vi "test_F9P_fgv-ver.vi"() -> ()   [LabVIEW 2019] (continued)
,2,13,08,65,355,35,09,07,194,,10,16,222,19,11,37,142,,3*73\r\n$GBGSV,4,3,13,13,50,315,36,14,76,037,37,28,59,310,,33,73,239,,3*78\r\n$GBGSV,4,4,13,34,13,142,,3*44\r\n$GNGLL,3723.61864,N,12656.97538,E,064330.00,A,A*7B\r\n$GNRMC,064331.00,A,3723.61873,N,12656.97627,E,2.634,76.09,250720,,,A,V*35\r\n$GNVTG,76.09,T,,M,2.634,N,4.879,K,A*1A\r\n$GNGGA,064331.00,3723.61873,N,12656.97627,E,1,12,0.67,43.8,M,18.5,M,,*75\r\n$GNGSA,A,3,17,19,06,12,05,02,09,,,,,,1.19,0.67,0.98,1*0D\r\n$GNGSA,A,3,85,70,71,72,,,,,,,,,1.19,0.67,0.98,2*02\r\n$GNGSA,A,3,36,19,11,04,09,12,,,,,,,1.19,0.67,0.98,3*09\r\n$GNGSA,A,3,28,14,13,33,08,10,,,,,,,1.19,0.67,0.98,4*09\r\n$GPGSV,4,1,13,02,66,335,45,04,08,037,40,05,48,262,42,06,58,077,45,1*6A\r\n$GPGSV,4,2,13,07,06,104,,09,38,057,48,12,18,263,,13,08,191,19,1*6E\r\n$GPGSV,4,3,13,17,19,158,28,19,37,161,33,25,11,294,20,29,07,323,16,1*60\r\n$GPGSV,4,4,13,30,01,134,,1*52\r\n$GPGSV,4,1,13,02,66,335,,04,08,037,39,05,48,262,37,06,58,077,39,6*6B\r\n$GPGSV,4,2,13,07,06,104,,09,38,057,42,12,18,263,12,13,08,191,,6*68\r\n$GPGSV,4,3,13,17,19,158,28,19,37,161,,25,11,294,,29,07,323,,6*62\r\n$GPGSV,4,4,13,30,01,134,,6*55\r\n$GLGSV,2,1,06,70,54,030,29,71,69,224,39,72,18,217,28,84,08,134,08,1*7C\r\n$GLGSV,2,2,06,85,63,113,37,86,52,337,,1*7F\r\n$GLGSV,2,1,06,70,54,030,,71,69,224,28,72,18,217,20,84,08,134,11,3*75\r\n$GLGSV,2,2,06,85,63,113,28,86,52,337,,3*73\r\n$GAGSV,3,1,09,02,04,287,08,04,68,085,43,09,44,196,25,11,78,037,40,7*74\r\n$GAGSV,3,2,09,12,32,115,29,18,55,284,40,19,17,042,31,25,01,241,,7*7F\r\n$GAGSV,3,3,09,36,35,314,22,7*4F\r\n$GAGSV,3,1,09,02,04,287,,04,68,085,39,09,44,196,22,11,78,037,32,2*76\r\n$GAGSV,3,2,09,12,32,115,25,18,55,284,43,19,17,042,31,25,01,241,,2*75\r\n$GAGSV,3,3,09,36,35,314,22,2*4A\r\n$GBGSV,4,1,13,04,35,133,,05,09,257,,06,27,182,,07,09,201,,1*7B\r\n$GBGSV,4,2,13,08,65,355,41,09,07,194,,10,16,222,19,11,37,142,,1*72\r\n$GBGSV,4,3,13,13,50,315,39,14,76,037,44,28,59,310,42,33,73,239,41,1*72\r\n$GBGSV,4,4,13,34,13,142,23,1*47\r\n$GBGSV,4,1,13,04,35,133,,05,09,257,,06,27,182,,07,09,201,17,3*7F\r\n$GBGSV,4,2,13,08,65,355,36,09,07,194,,10,16,222,19,11,37,142,,3*70\r\n$GBGSV,4,3,13,13,50,315,38,14,76,037,39,28,59,310,,33,73,239,,3*78\r\n$GBGSV,4,4,13,34,13,142,,3*44\r\n$GNGLL,3723.61873,N,12656.97627,E,064331.00,A,A*71\r\n$GNRMC,064332.00,A,3723.61883,N,12656.97715,E,2.685,76.91,250720,,,A,V*32\r\n$GNVTG,76.91,T,,M,2.685,N,4.973,K,A*1A\r\n$GNGGA,064332.00,3723.61883,N,12656.97715,E,1,12,0.67,43.7,M,18.5,M,,*76\r\n$GNGSA,A,3,17,19,06,12,05,02,09,,,,,,1.19,0.67,0.98,1*0D\r\n$GNGSA,A,3,85,70,71,72,,,,,,,,,1.19,0.67,0.98,2*02\r\n$GNGSA,A,3,36,19,11,04,09,12,,,,,,,1.19,0.67,0.98,3*09\r\n$GNGSA,A,3,28,34,14,13,33,08,10,,,,,,1.19,0.67,0.98,4*0E\r\n$GPGSV,4,1,13,02,66,335,45,04,08,037,27,05,48,262,43,06,58,077,43,1*6C\r\n$GPGSV,4,2,13,07,06,104,,09,38,057,45,12,18,263,,13,08,191,22,1*6B\r\n$GPGSV,4,3,13,17,19,158,33,19,37,161,28,25,11,294,19,29,07,323,17,1*6B\r\n$GPGSV,4,4,13,30,01,134,,1*52\r\n$GPGSV,4,1,13,02,66,335,,04,08,037,37,05,48,262,38,06,58,077,38,6*6B\r\n$GPGSV,4,2,13,07,06,104,,09,38,057,43,12,18,263,11,13,08,191,,6*6A\r\n$GPGSV,4,3,13,17,19,158,29,19,37,161,,25,11,294,,29,07,323,,6*63\r\n$GPGSV,4,4,13,30,01,134,,6*55\r\n$GLGSV,2,1,06,70,54,030,36,71,69,224,40,72,18,217,30,84,08,134,09,1*74\r\n$GLGSV,2,2,06,85,63,113,30,86,52,337,,1*78\r\n$GLGSV,2,1,06,70,54,030,,71,69,224,28,72,18,217,20,84,08,134,11,3*75\r\n$GLGSV,2,2,06,85,63,113,28,86,52,337,,3*73\r\n$GAGSV,3,1,09,02,04,287,10,04,68,085,40,09,44,196,32,11,78,037,38,7*77\r\n$GAGSV,3,2,09,12,32,115,29,18,55,284,41,19,17,042,33,25,01,241,,7*7C\r\n$GAGSV,3,3,09,36,35,314,24,7*49\r\n$GAGSV,3,1,09,02,04,287,,04,68,085,35,09,44,196,29,11,78,037,31,2*72\r\n$GAGSV,3,2,09,12,32,115,25,18,55,284,44,19,17,042,37,25,01,241,,2*74\r\n$GAGSV,3,3,09,36,35,314,22,2*4A\r\n$GBGSV,4,1,13,04,35,133,,05,09,257,,06,27,182,,07,09,201,,1*7B\r\n$GBGSV,4,2,13,08,65,355,41,09,07,194,,10,16,222,19,11,37,142,,1*72\r\n$GBGSV,4,3,13,13,50,315,39,14,76,037,42,28,59,310,43,33,73,239,41,1*75\r\n$GBGSV,4,4,13,34,13,142,25,1*41\r\n$GBGSV,4,1,13,04,35,133,,05,09,257,,06,27,182,,07,09,201,13,3*7B\r\n$GBGSV,4,2,13,08,65,355,36,09,07,194,,10,16,222,21,11,37,142,,3*7B\r\n$GBGSV,4,3,13,13,50,315,35,14,76,037,37,28,59,310,,33,73,239,,3*7B\r\n$GBGSV,4,4,13,34,13,142,,3*44\r\n$GNGLL,3723.61883,N,12656.97715,E,064332.00,A,A*7D\r\n$GNRMC,064333.00,A,3723.61900,N,12656.97803,E,2.812,70.91,250720,,,A,V*37\r\n$GNVTG,70.91,T,,M,2.812,N,5.207,K,A*15\r\n$GNGGA,064333.00,3723.61900,N,12656.97803,E,1,12,0.67,43.7,M,18.5,M,,*75\r\n$GNGSA,A,3,17,19,06,05,02,09,,,,,,,1.18,0.67,0.98,1*0F\r\n$GNGSA,A,3,85,70,71,72,,,,,,,,,1.18,0.67,0.98,2*03\r\n$GNGSA,A,3,36,19,11,04,09,12,,,,,,,1.18,0.67,0.98,3*08\r\n$GNGSA,A,3,28,11,14,13,33,08,10,,,,,,1.18,0.67,0.98,4*08\r\n$GPGSV,4,1,13,02,66,335,44,04,08,037,37,05,48,262,42,06,58,077,46,1*68\r\n$GPGSV,4,2,13,07,06,104,,09,38,057,45,12,18,263,,13,08,191,21,1*68\r\n$GPGSV,4,3,13,17,19,158,29,19,37,161,32,25,11,294,20,29,07,323,15,1*63\r\n$GPGSV,4,4,13,30,01,134,,1*52\r\n$GPGSV,4,1,13,02,66,335,,04,08,037,37,05,48,262,38,06,58,077,37,6*64\r\n$GPGSV,4,2,13,07,06,104,,09,38,057,43,12,18,263,,13,08,191,,6*6A\r\n$GPGSV,4,3,13,17,19,158,26,19,37,161,,25,11,294,,29,07,323,,6*6C\r\n$GPGSV,4,4,13,30,01,134,,6*55\r\n$GLGSV,2,1,06,70,54,030,35,71,69,224,42,72,18,217,30,84,08,134,15,1*78\r\n$GLGSV,2,2,06,85,63,113,41,86,52,337,,1*7E\r\n$GLGSV,2,1,06,70,54,030,,71,69,224,27,72,18,217,19,84,08,134,10,3*71\r\n$GLGSV,2,2,06,85,63,113,28,86,52,337,,3*73\r\n$GAGSV,3,1,09,02,04,287,08,04,68,085,43,09,44,196,36,11,78,037,40,7*76\r\n$GAGSV,3,2,09,12,32,115,31,18,55,284,41,19,17,042,34,25,01,241,,7*72\r\n$GAGSV,3,3,09,36,35,314,24,7*49\r\n$GAGSV,3,1,09,02,04,287,,04,68,085,37,09,44,196,33,11,78,037,33,2*79\r\n$GAGSV,3,2,09,12,32,115,24,18,55,284,45,19,17,042,37,25,01,241,,2*74\r\n$GAGSV,3,3,09,36,35,314,23,2*4B\r\n$GBGSV,4,1,13,04,35,133,,05,09,257,,06,27,182,,07,09,201,,1*7B\r\n$GBGSV,4,2,13,08,65,355,41,09,07,194,,10,16,222,18,11,37,142,30,1*70\r\n$GBGSV,4,3,13,13,50,315,40,14,76,037,44,28,59,310,42,33,73,239,42,1*7F\r\n$GBGSV,4,4,13,34,13,142,,1*46\r\n$GBGSV,4,1,13,04,35,133,,05,09,257,,06,27,182,,07,09,201,14,3*7C\r\n$GBGSV,4,2,13,08,65,355,38,09,07,194,,10,16,222,20,11,37,142,,3*74\r\n$GBGSV,4,3,13,13,50,315,38,14,76,037,37,28,59,310,,33,73,239,,3*76\r\n$GBGSV,4,4,13,34,13,142,,3*44\r\n$GNGLL,3723.61900,N,12656.97803,E,064333.00,A,A*7E\r\n$GNRMC,064334.00,A,3723.61923,N,12656.97890,E,2.813,67.43,250720,,,A,V*33\r\n$GNVTG,67.43,T,,M,2.813,N,5.210,K,A*1B\r\n$GNGGA,064334.00,3723.61923,N,12656.97890,E,1,12,0.66,43.6,M,18.5,M,,*79\r\n$GNGSA,A,3,17,19,06,05,02,09,,,,,,,1.18,0.66,0.98,1*0E\r\n$GNGSA,A,3,85,70,71,72,,,,,,,,,1.18,0.66,0.98,2*02\r\n$GNGSA,A,3,36,19,11,04,09,12,,,,,,,1.18,0.66,0.98,3*09\r\n$GNGSA,A,3,28,11,14,13,33,08,10,,,,,,1.18,0.66,0.98,4*09\r\n$GPGSV,4,1,13,02,66,335,43,04,08,037,33,05,48,262,41,06,58,077,49,1*67\r\n$GPGSV,4,2,13,07,06,104,,09,38,057,40,12,18,263,,13,08,191,20,1*6C\r\n$GPGSV,4,3,13,17,19,158,34,19,37,161,28,25,11,294,20,29,07,323,16,1*67\r\n$GPGSV,4,4,13,30,01,134,,1*52\r\n$GPGSV,4,1,13,02,66,335,,04,08,037,32,05,48,262,37,06,58,077,32,6*6B\r\n$GPGSV,4,2,13,07,06,104,,09,38,057,40,12,18,263,,13,08,191,,6*69\r\n$GPGSV,4,3,13,17,19,158,31,19,37,161,,25,11,294,,29,07,323,,6*6A\r\n$GPGSV,4,4,13,30,01,134,,6*55\r\n$GLGSV,2,1,06,70,54,030,27,71,69,224,42,72,18,217,30,84,08,134,12,1*7C\r\n$GLGSV,2,2,06,85,63,113,43,86,52,337,,1*7C\r\n$GLGSV,2,1,06,70,54,030,,71,69,224,28,72,18,217,19,84,08,134,10,3*7E\r\n$GLGSV,2,2,06,85,63,113,27,86,52,337,,3*7C\r\n$GAGSV,3,1,09,02,04,287,11,04,68,085,45,09,44,196,38,11,78,037,38,7*79\r\n$GAGSV,3,2,09,12,32,115,25,18,55,284,38,19,17,042,34,25,01,241,,7*79\r\n$GAGSV,3,3,09,36,35,314,25,7*48\r\n$GAGSV,3,1,09,02,04,287,,04,68,085,37,09,44,196,36,11,78,037,35,2*7A\r\n$GAGSV,3,2,09,12,32,115,24,18,55,284,44,19,17,042,35,25,01,241,,2*77\r\n$GAGSV,3,3,09,36,35,314,23,2*4B\r\n$GBGSV,4,1,13,04,35,133,,05,09,257,,06,27,182,,07,09,201,,1*7B\r\n$GBGSV,4,2,13,08,65,355,41,09,07,194,,10,16,222,18,11,37,142,34,1*74\r\n$GBGSV,4,3,13,13,50,315,39,14,76,037,44,28,59,310,41,33,73,239,42,1*72\r\n$GBGSV,4,4,13,34,13,142,,1*46\r\n$GBGSV,4,1,13,04,35,133,,05,09,257,,06,27,182,,07,09,201,,3*79\r\n$GBGSV,4,2,13,08,65,355,38,09,07,194,,10,16,222,21,11,37,142,,3*75\r\n$GBGSV,4,3,13,13,50,315,39,14,76,037,38,28,59,310,,33,73,239,,3*78\r\n$GBGSV,4,4,13,34,13,142,,3*44\r\n$GNGLL,3723.61923,N,12656.97890,E,064334.00,A,A*72\r\n$GNRMC,064335.00,A,3723.61955,N,12656.97980,E,3.032,64.24,250720,,,A,V*3B\r\n$GNVTG,64.24,T,,M,3.032,N,5.615,K,A*12\r\n$GNGGA,064335.00,3723.61955,N,12656.97980,E,1,12,0.66,44.0,M,18.5,M,,*78\r\n$GNGSA,A,3,17,19,06,05,02,09,,,,,,,1.18,0.66,0.98,1*0E\r\n$GNGSA,A,3,85,70,71,72,,,,,,,,,1.18,0.66,0.98,2*02\r\n$GNGSA,A,3,36,19,11,04,09,12,,,,,,,1.18,0.66,0.98,3*09\r\n$GNGSA,A,3,28,11,14,13,33,08,10,,,,,,1.18,0.66,0.98,4*09\r\n$GPGSV,4,1,13,02,66,335,40,04,08,037,30,05,48,262,41,06,58,077,49,1*67\r\n$GPGSV,4,2,13,07,06,104,,09,38,057,42,12,18,262,,13,08,191,20,1*6F\r\n$GPGSV,4,3,13,17,19,158,32,19,37,161,29,25,11,294,20,29,07,323,16,1*60\r\n$GPGSV,4,4,13,30,01,134,,1*52\r\n$GPGSV,4,1,13,02,66,335,,04,08,037,35,05,48,262,35,06,58,077,35,6*69\r\n$GPGSV,4,2,13,07,06,104,,09,38,057,43,12,18,262,,13,08,191,,6*6B\r\n$GPGSV,4,3,13,17,19,158,27,19,37,161,,25,11,294,,29,07,323,,6*6D\r\n$GPGSV,4,4,13,30,01,134,,6*55\r\n$GLGSV,2,1,06,70,54,030,32,71,69,224,42,72,18,217,29,84,08,134,09,1*7A\r\n$GLGSV,2,2,06,85,63,113,40,86,52,337,,1*7F\r\n$GLGSV,2,1,06,70,54,030,,71,69,224,29,72,18,217,20,84,08,134,15,3*70\r\n$GLGSV,2,2,06,85,63,113,26,86,52,337,,3*7D\r\n$GAGSV,3,1,09,02,04,287,08,04,68,085,45,09,44,196,38,11,78,037,39,7*70\r\n$GAGSV,3,2,09,12,32,115,35,18,55,284,39,19,17,042,39,25,01,241,,7*74\r\n$GAGSV,3,3,09,36,35,314,24,7*49\r\n$GAGSV,3,1,09,02,04,287,,04,68,085,37,09,44,196,34,11,78,037,32,2*7F\r\n$GAGSV,3,2,09,12,32,115,22,18,55,284,44,19,17,042,34,25,01,241,,2*70\r\n$GAGSV,3,3,09,36,35,314,23,2*4B\r\n$GBGSV,4,1,13,04,35,133,,05,09,257,,06,27,182,,07,09,201,,1*7B\r\n$GBGSV,4,2,13,08,65,355,40,09,07,194,,10,16,222,21,11,37,142,29,1*73\r\n$GBGSV,4,3,13,13,50,315,39,14,76,037,44,28,59,310,41,33,73,239,42,1*72\r\n$GBGSV,4,4,13,34,13,142,,1*46\r\n$GBGSV,4,1,13,04,35,133,,05,09,257,,06,27,182,,07,09,201,,3*79\r\n$GBGSV,4,2,13,08,65,355,38,09,07,194,,10,16,222,21,11,37,142,28,3*7F\r\n$GBGSV,4,3,13,13,50,315,37,14,76,037,39,28,59,310,,33,73,239,,3*77\r\n$GBGSV,4,4,13,34,13,142,,3*44\r\n$GNGLL,3723.61955,N,12656.97980,E,064335.00,A,A*72\r\n$GNRMC,064336.00,A,3723.61979,N,12656.98066,E,2.704,64.77,250720,,,A,V*3D\r\n$GNVTG,64.77,T,,M,2.704,N,5.008,K,A*1D\r\n$GNGGA,064336.00,3723.61979,N,12656.98066,E,1,12,0.66,43.8,M,18.5,M,,*74\r\n$GNGSA,A,3,17,19,06,05,02,09,,,,,,,1.18,0.66,0.98,1*0E\r\n$GNGSA,A,3,85,70,71,72,,,,,,,,,1.18,0.66,0.98,2*02\r\n$GNGSA,A,3,36,19,11,04,09,12,,,,,,,1.18,0.66,0.98,3*09\r\n$GNGSA,A,3,28,11,14,13,33,08,10,,,,,,1.18,0.66,0.98,4*09\r\n$GPGSV,4,1,13,02,66,335,41,04,08,037,34,05,48,262,38,06,58,077,46,1*63\r\n$GPGSV,4,2,13,07,06,104,,09,38,057,44,12,18,262,,13,09,191,20,1*68\r\n$GPGSV,4,3,13,17,19,158,31,19,37,161,30,25,11,294,21,29,07,323,17,1*6B\r\n$GPGSV,4,4,13,30,01,134,,1*52\r\n$GPGSV,4,1,13,02,66,335,,04,08,037,30,05,48,262,36,06,58,077,38,6*62\r\n$GPGSV,4,2,13,07,06,104,,09,38,057,43,12,18,262,19,13,09,191,,6*62\r\n$GPGSV,4,3,13,17,19,158,27,19,37,161,,25,11,294,,29,07,323,,6*6D\r\n$GPGSV,4,4,13,30,01,134,,6*55\r\n$GLGSV,2,1,06,70,54,030,28,71,69,224,40,72,18,217,22,84,08,134,09,1*78\r\n$GLGSV,2,2,06,85,63,113,36,86,52,337,,1*7E\r\n$GLGSV,2,1,06,70,54,030,,71,69,224,28,72,18,217,20,84,08,134,17,3*73\r\n$GLGSV,2,2,06,85,63,113,26,86,52,337,,3*7D\r\n$GAGSV,3,1,09,02,04,287,08,04,68,085,44,09,44,196,40,11,78,037,40,7*70\r\n$GAGSV,3,2,09,12,32,115,35,18,55,284,41,19,17,042,40,25,01,241,,7*75\r\n$GAGSV,3,3,09,36,35,314,24,7*49\r\n$GAGSV,3,1,09,02,04,287,,04,68,085,37,09,44,196,37,11,78,037,32,2*7C\r\n$GAGSV,3,2,09,12,32,115,23,18,55,284,44,19,17,042,35,25,01,241,,2*70\r\n$GAGSV,3,3,09,36,35,314,25,2*4D\r\n$GBGSV,4,1,13,04,35,133,,05,09,257,,06,27,182,,07,09,201,,1*7B\r\n$GBGSV,4,2,13,08,65,355,42,09,07,194,,10,16,222,21,11,37,142,29,1*71\r\n$GBGSV,4,3,13,13,50,315,41,14,76,037,45,28,59,310,42,33,73,239,43,1*7E\r\n$GBGSV,4,4,13,34,13,142,,1*46\r\n$GBGSV,4,1,13,04,35,133,,05,09,257,,06,27,182,,07,09,201,,3*79\r\n$GBGSV,4,2,13,08,65,355,37,09,07,194,,10,16,222,23,11,37,142,26,3*7C\r\n$GBGSV,4,3,13,13,50,315,39,14,76,037,39,28,59,310,,33,73,239,,3*79\r\n$GBGSV,4,4,13,34,13,142,,3*44\r\n$GNGLL,3723.61979,N,12656.98066,E,064336.00,A,A*71\r\n$GNRMC,064337.00,A,3723.62002,N,12656.98152,E,2.800,65.01,250720,,,A,V*37\r\n$GNVTG,65.01,T,,M,2.800,N,5.185,K,A*12\r\n$GNGGA,064337.00,3723.62002,N,12656.98152,E,1,12,0.66,43.6,M,18.5,M,,*7B\r\n$GNGSA,A,3,17,19,06,05,02,09,,,,,,,1.18,0.66,0.98,1*0E\r\n$GNGSA,A,3,85,70,71,72,,,,,,,,,1.18,0.66,0.98,2*02\r\n$GNGSA,A,3,36,19,11,04,09,12,,,,,,,1.18,0.66,0.98,3*09\r\n$GNGSA,A,3,28,11,14,13,33,08,10,,,,,,1.18,0.66,0.98,4*09\r\n$GPGSV,4,1,13,02,66,335,42,04,08,037,37,05,48,262,38,06,58,077,46,1*63\r\n$GPGSV,4,2,13,07,06,104,,09,38,057,44,12,18,262,,13,09,191,19,1*62\r\n$GPGSV,4,3,13,17,19,158,31,19,37,161,30,25,11,294,21,29,07,323,17,1*6B\r\n$GPGSV,4,4,13,30,01,134,,1*52\r\n$GPGSV,4,1,13,02,66,335,,04,08,037,22,05,48,262,38,06,58,077,37,6*60\r\n$GPGSV,4,2,13,07,06,104,,09,38,057,43,12,18,262,17,13,09,191,,6*6C\r\n$GPGSV,4,3,13,17,19,158,28,19,37,161,,25,11,294,,29,07,323,,6*62\r\n$GPGSV,4,4,13,30,01,134,,6*55\r\n$GLGSV,2,1,06,70,54,030,29,71,69,224,41,72,18,217,29,84,08,134,08,1*72\r\n$GLGSV,2,2,06,85,63,113,36,86,52,337,,1*7E\r\n$GLGSV,2,1,06,70,54,030,,71,69,224,28,72,18,217,20,84,08,134,17,3*73\r\n$GLGSV,2,2,06,85,63,113,26,86,52,337,,3*7D\r\n$GAGSV,3,1,09,02,04,287,06,04,68,085,43,09,44,196,40,11,78,037,40,7*79\r\n$GAGSV,3,2,09,12,32,115,24,18,55,284,41,19,17,042,35,25,01,241,,7*77\r\n$GAGSV,3,3,09,36,35,314,30,7*4C\r\n$GAGSV,3,1,09,02,04,287,,04,68,085,37,09,44,196,36,11,78,037,31,2*7E\r\n$GAGSV,3,2,09,12,32,115,24,18,55,284,43,19,17,042,36,25,01,241,,2*73\r\n$GAGSV,3,3,09,36,35,314,26,2*4E\r\n$GBGSV,4,1,13,04,35,133,,05,09,257,,06,27,182,,07,09,201,,1*7B\r\n$GBGSV,4,2,13,08,65,355,41,09,07,194,,10,16,222,20,11,37,142,29,1*73\r\n$GBGSV,4,3,13,13,50,315,41,14,76,037,44,28,59,310,42,33,73,239,41,1*7D\r\n$GBGSV,4,4,13,34,13,142,,1*46\r\n$GBGSV,4,1,13,04,35,133,,05,09,257,,06,27,182,,07,09,201,,3*79\r\n$GBGSV,4,2,13,08,65,355,36,09,07,194,,10,16,222,24,11,37,142,34,3*79\r\n$GBGSV,4,3,13,13,50,315,39,14,76,037,38,28,59,310,,33,73,239,,3*78\r\n$GBGSV,4,4,13,34,13,142,,3*44\r\n$GNGLL,3723.62002,N,12656.98152,E,064337.00,A,A*70\r\n$GNRMC,064338.00,A,3723.62025,N,12656.98244,E,2.944,65.53,250720,,,A,V*3F\r\n$GNVTG,65.53,T,,M,2.944,N,5.452,K,A*1B\r\n$GNGGA,064338.00,3723.62025,N,12656.98244,E,1,12,0.66,43.3,M,18.5,M,,*70\r\n$GNGSA,A,3,17,19,06,05,02,09,,,,,,,1.18,0.66,0.98,1*0E\r\n$GNGSA,A,3,85,70,71,72,,,,,,,,,1.18,0.66,0.98,2*02\r\n$GNGSA,A,3,36,19,11,04,09,12,,,,,,,1.18,0.66,0.98,3*09\r\n$GNGSA,A,3,28,11,14,13,33,08,10,,,,,,1.18,0.66,0.98,4*09\r\n$GPGSV,4,1,13,02,66,335,43,04,08,037,42,05,48,262,37,06,58,077,48,1*61\r\n$GPGSV,4,2,13,07,06,104,,09,38,057,40,12,18,262,,13,09,191,,1*6E\r\n$GPGSV,4,3,13,17,19,158,30,19,37,161,30,25,11,294,23,29,07,323,18,1*67\r\n$GPGSV,4,4,13,30,01,134,,1*52\r\n$GPGSV,4,1,13,02,66,335,,04,08,037,29,05,48,262,38,06,58,077,37,6*6B\r\n$GPGSV,4,2,13,07,06,104,,09,38,057,41,12,18,262,16,13,09,191,,6*6F\r\n$GPGSV,4,3,13,17,19,158,28,19,37,161,,25,11,294,24,29,07,323,,6*64\r\n$GPGSV,4,4,13,30,01,134,,6*55\r\n$GLGSV,2,1,06,70,54,030,28,71,69,224,41,72,18,217,23,84,08,134,07,1*76\r\n$GLGSV,2,2,06,85,63,113,39,86,52,337,,1*71\r\n$GLGSV,2,1,06,70,54,030,,71,69,224,28,72,18,217,20,84,08,134,12,3*76\r\n$GLGSV,2,2,06,85,63,113,26,86,52,337,,3*7D\r\n$GAGSV,3,1,09,02,04,287,08,04,68,085,45,09,44,196,39,11,78,037,39,7*71\r\n$GAGSV,3,2,09,12,32,115,32,18,55,284,38,19,17,042,32,25,01,241,,7*79\r\n$GAGSV,3,3,09,36,35,314,34,7*48\r\n$GAGSV,3,1,09,02,04,287,,04,68,085,37,09,44,196,37,11,78,037,32,2*7C\r\n$GAGSV,3,2,09,12,32,115,32,18,55,284,43,19,17,042,36,25,01,241,,2*74\r\n$GAGSV,3,3,09,36,35,314,32,2*4B\r\n$GBGSV,4,1,13,04,35,133,,05,09,257,,06,27,182,,07,09,201,,1*7B\r\n$GBGSV,4,2,13,08,65,355,40,09,07,194,,10,16,222,19,11,37,142,28,1*79\r\n$GBGSV,4,3,13,13,50,315,40,14,76,037,45,28,59,310,42,33,73,239,41,1*7D\r\n$GBGSV,4,4,13,34,13,142,,1*46\r\n$GBGSV,4,1,13,04,35,133,,05,09,257,,06,27,182,,07,09,201,,3*79\r\n$GBGSV,4,2,13,08,65,355,36,09,07,194,,10,16,222,21,11,37,142,,3*7B\r\n$GBGSV,4,3,13,13,50,315,37,14,76,037,38,28,59,310,,33,73,239,,3*76\r\n$GBGSV,4,4,13,34,13,142,,3*44\r\n$GNGLL,3723.62025,N,12656.98244,E,064338.00,A,A*7E\r\n$GNRMC,064339.00,A,3723.62051,N,12656.98334,E,2.929,64.74,250720,,,A,V*34\r\n$GNVTG,64.74,T,,M,2.929,N,5.424,K,A*15\r\n$GNGGA,064339.00,3723.62051,N,12656.98334,E,1,12,0.67,43.0,M,18.5,M,,*76\r\n$GNGSA,A,3,17,19,06,05,02,09,,,,,,,1.19,0.67,0.98,1*0E\r\n$GNGSA,A,3,85,70,71,72,,,,,,,,,1.19,0.67,0.98,2*02\r\n$GNGSA,A,3,36,19,11,04,09,12,,,,,,,1.19,0.67,0.98,3*09\r\n$GNGSA,A,3,28,14,13,33,08,10,,,,,,,1.19,0.67,0.98,4*09\r\n$GPGSV,4,1,13,02,66,335,45,04,08,037,44,05,48,262,38,06,58,077,47,1*61\r\n$GPGSV,4,2,13,07,06,104,21,09,38,057,42,12,18,262,,13,09,191,,1*6F\r\n$GPGSV,4,3,13,17,18,158,30,19,37,161,33,25,11,294,24,29,07,323,19,1*63\r\n$GPGSV,4,4,13,30,01,134,,1*52\r\n$GPGSV,4,1,13,02,66,335,,04,08,037,34,05,48,262,37,06,58,077,40,6*68\r\n$GPGSV,4,2,13,07,06,104,,09,38,057,39,12,18,262,16,13,09,191,,6*60\r\n$GPGSV,4,3,13,17,18,158,27,19,37,161,,25,11,294,23,29,07,323,,6*6D\r\n$GPGSV,4,4,13,30,01,134,,6*55\r\n$GLGSV,2,1,06,70,54,030,35,71,69,224,40,72,18,217,24,84,08,134,10,1*7A\r\n$GLGSV,2,2,06,85,63,113,39,86,52,337,,1*71\r\n$GLGSV,2,1,06,70,54,030,,71,69,224,28,72,18,217,18,84,08,134,13,3*7C\r\n$GLGSV,2,2,06,85,63,113,26,86,52,337,,3*7D\r\n$GAGSV,3,1,09,02,04,287,09,04,68,085,41,09,44,196,42,11,78,037,41,7*77\r\n$GAGSV,3,2,09,12,32,115,37,18,55,284,42,19,17,042,36,25,01,241,,7*75\r\n$GAGSV,3,3,09,36,35,314,33,7*4F\r\n$GAGSV,3,1,09,02,04,287,,04,68,085,36,09,44,196,37,11,78,037,31,2*7E\r\n$GAGSV,3,2,09,12,32,115,25,18,55,284,44,19,17,042,30,25,01,241,,2*73\r\n$GAGSV,3,3,09,36,35,314,32,2*4B\r\n$GBGSV,4,1,13,04,35,133,,05,09,257,,06,27,182,,07,09,201,,1*7B\r\n$GBGSV,4,2,13,08,65,355,40,09,07,194,,10,16,222,21,11,37,142,,1*78\r\n$GBGSV,4,3,13,13,50,315,40,14,76,037,45,28,59,310,43,33,73,239,42,1*7F\r\n$GBGSV,4,4,13,34,13,142,,1*46\r\n$GBGSV,4,1,13,04,35,133,,05,09,257,,06,27,182,,07,09,201,,3*79\r\n$GBGSV,4,2,13,08,65,355,34,09,07,194,,10,16,222,21,11,37,142,,3*79\r\n$GBGSV,4,3,13,13,50,315,37,14,76,037,40,28,59,310,,33,73,239,,3*79\r\n$GBGSV,4,4,13,34,13,142,,3*44\r\n$GNGLL,3723.62051,N,12656.98334,E,064339.00,A,A*7A\r\n$GNRMC,064340.00,A,3723.62075,N,12656.98429,E,2.948,68.00,250720,,,A,V*3F\r\n$GNVTG,68.00,T,,M,2.948,N,5.459,K,A*17\r\n$GNGGA,064340.00,3723.62075,N,12656.98429,E,1,12,0.63,43.1,M,18.5,M,,*70\r\n$GNGSA,A,3,17,19,06,12,05,02,09,,,,,,1.10,0.63,0.90,1*08\r\n$GNGSA,A,3,85,70,71,72,,,,,,,,,1.10,0.63,0.90,2*07\r\n$GNGSA,A,3,36,19,11,04,09,12,,,,,,,1.10,0.63,0.90,3*0C\r\n$GNGSA,A,3,28,14,13,33,08,10,,,,,,,1.10,0.63,0.90,4*0C\r\n$GPGSV,4,1,13,02,66,335,45,04,08,037,37,05,48,262,43,06,58,077,47,1*69\r\n$GPGSV,4,2,13,07,06,104,,09,38,057,43,12,18,262,20,13,09,191,23,1*6E\r\n$GPGSV,4,3,13,17,18,158,29,19,37,161,23,25,11,294,23,29,07,323,19,1*6D\r\n$GPGSV,4,4,13,30,01,134,,1*52\r\n$GPGSV,4,1,13,02,66,335,,04,08,037,29,05,48,262,38,06,58,077,34,6*68\r\n$GPGSV,4,2,13,07,06,104,,09,38,057,39,12,18,262,17,13,09,191,,6*61\r\n$GPGSV,4,3,13,17,18,158,26,19,37,161,,25,11,294,23,29,07,323,21,6*6F\r\n$GPGSV,4,4,13,30,01,134,,6*55\r\n$GLGSV,2,1,06,70,54,030,32,71,69,224,41,72,18,217,30,84,08,134,13,1*7A\r\n$GLGSV,2,2,06,85,63,113,44,86,52,337,,1*7B\r\n$GLGSV,2,1,06,70,54,030,,71,69,224,31,72,18,217,17,84,08,134,17,3*7F\r\n$GLGSV,2,2,06,85,63,113,26,86,52,337,,3*7D\r\n$GAGSV,3,1,09,02,04,287,09,04,68,085,46,09,44,196,39,11,78,037,41,7*7C\r\n$GAGSV,3,2,09,12,32,115,33,18,55,284,40,19,
